vi "macro_Ramsete_Execute_External_Odometry_ENG.vi"() -> ()   [LabVIEW 2019, in "Trajectory_Library.lvlib"]
uses:
  Trajectory_Library.lvlib
  TypeDef/TRANSLATION2D.ctl
  TypeDef/ROTATION2D.ctl
  TypeDef/POSE2D.ctl
  TypeDef/TRAJ_STATE.ctl
panel:
  out "Right Speed Dmd FT/S":dbl
  out "Left Speed Dmd FT/S":dbl
  in  "Current Pose ENG":T1 {"ROTATION"."SIN" format="%13.4f"; "ROTATION"."COS" format="%13.4f"; "ROTATION"."VALUE" format="%13.4f"; "TRANSLATION"."Y" format="%14.3f"; "TRANSLATION"."X" format="%14.3f"}
  in  "TRAJ_STATE SI":T4 {"POSE"."ROTATION"."SIN" format="%13.4f"; "POSE"."ROTATION"."COS" format="%13.4f"; "POSE"."ROTATION"."VALUE" format="%13.4f"; "POSE"."TRANSLATION"."Y" format="%14.3f"; "POSE"."TRANSLATION"."X" format="%14.3f"}
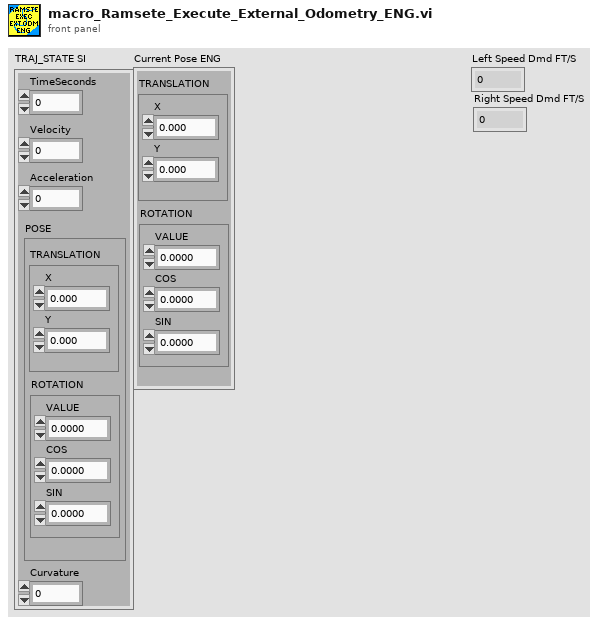
[diagram p1: front panel]
types:
  T1 = typedef "Trajectory_Library.lvlib/POSE2D.ctl" = cluster{"TRANSLATION":T2, "ROTATION":T3}
  T2 = typedef "Trajectory_Library.lvlib/TRANSLATION2D.ctl" = cluster{"X":dbl, "Y":dbl}
  T3 = typedef "Trajectory_Library.lvlib/ROTATION2D.ctl" = cluster{"VALUE":dbl, "COS":dbl, "SIN":dbl}
  T4 = typedef "Trajectory_Library.lvlib/TRAJ_STATE.ctl" = cluster{"TimeSeconds":dbl, "Velocity":dbl, "Acceleration":dbl, "POSE":T1, "Curvature":dbl}
  T5 = typedef "Trajectory_Library.lvlib/RAMSETE_EXE_TUNING.ctl" = cluster{"B":dbl, "Zeta":dbl, "X Tolerance M":dbl, "Y Tolerance M":dbl, "Heading Tolerance RAD":dbl, "Track Width M":dbl, "Max Speed M/S":dbl}
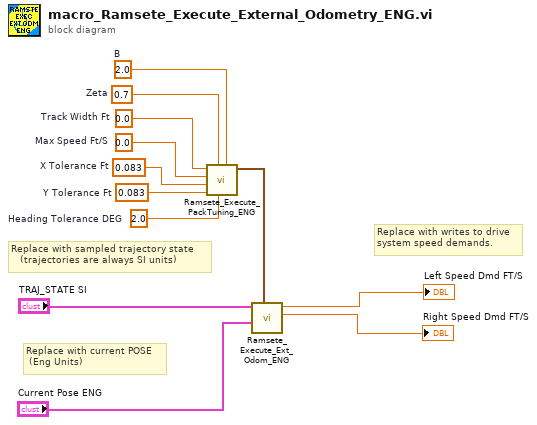
[diagram p0: block diagram]
diagram:
  w5 = 0.0  # Track Width Ft
  w6 = 0.0  # Max Speed Ft/S
  w7 = 0.083  # X Tolerance Ft
  w8 = 0.083  # Y Tolerance Ft
  w9 = 0.7  # Zeta
  w10 = 2.0  # Heading Tolerance DEG
  w11 = 2.0  # B
  # "Replace with writes to drive\nsystem speed demands."
  # "Replace with current POSE\n (Eng Units)"
  # "Replace with sampled trajectory state \n   (trajectories are always SI units)"
  n1 = call "Ramsete_Execute_PackTuning_ENG.vi"("B"=w11, "Heading Tolerance DEG"=w10, "Zeta"=w9, "Y Tolerance Ft"=w8, "X Tolerance Ft"=w7, "Max Speed Ft/S"=w6, "Track Width Ft"=w5) -> ("RAMSETE_EXE_TUNING"=w12:T5)  [unwired: 4 in]
  n2 = call "Ramsete_Execute_Ext_Odom_ENG.vi"("RAMSETE_EXE_TUNING SI"=w12, "Current Pose ENG"="Current Pose ENG", "TRAJ_STATE SI"="TRAJ_STATE SI") -> ("Right Speed Dmd FT/S"=→"Right Speed Dmd FT/S":dbl, "Left Speed Dmd FT/S"=→"Left Speed Dmd FT/S":dbl)  [unwired: 5 in, 2 out]
